vi "gearMiddlePeg.vi"   [LabVIEW 2016]
uses:
  <vilib>/Rock Robotics/WPI/Solenoid/WPI_SolenoidValue.ctl
  <vilib>/Rock Robotics/WPI/Solenoid/WPI_SolenoidSetEnum.vi
types:
  T1 = typedef "WPI_SolenoidValue.ctl" = enum16{"Off", "On", "Forward", "Reverse"}
  T2 = typedef "WPI_MotorControlDeviceRef.ctl" = cluster{"DeviceStatus":errorcluster, "Type":T3, "PWM":cluster{"PWM Channel":T4, "DeadBand":T5}, "CAN":cluster{"Device Number":u8, "SetOutput VI Ref":variant, "GetOutput VI Ref":variant, "Enable VI Ref":variant, "Disable VI Ref":variant, "Data":variant}, "Invert":bool}
  T3 = typedef "WPI_MotorControlType.ctl" = enum16{"PWM", "CAN"}
  T4 = typedef "FPGA_DIOPWMChannel.ctl" = enum8{"PWM 0", "PWM 1", "PWM 2", "PWM 3", "PWM 4", "PWM 5", "PWM 6", "PWM 7", "PWM 8", "PWM 9", "PWM MXP 0", "PWM MXP 1", "PWM MXP 2", "PWM MXP 3", "PWM MXP 4", "PWM MXP 5", "PWM MXP 6", "PWM MXP 7", "PWM MXP 8", "PWM MXP 9", "Invalid"}
  T5 = typedef "WPI_PWMDeadband.ctl" = cluster{"Name":string, "maxPositivePwm":i32, "minPositivePwm":i32, "centerPwm":i32, "maxNegativePwm":i32, "minNegativePwm":i32, "angularRange":u16}
  T6 = typedef "WPI_SolenoidDevRef.ctl" = cluster{"DevStatus":errorcluster, "Pneumatics Control Module":u8, "Forward Solenoid Channel":T7, "Reverse Solenoid Channel":T7}
  T7 = typedef "WPI_SolenoidChannel.ctl" = enum8{"Solenoid 0", "Solenoid 1", "Solenoid 2", "Solenoid 3", "Solenoid 4", "Solenoid 5", "Solenoid 6", "Solenoid 7", "Invalid"}
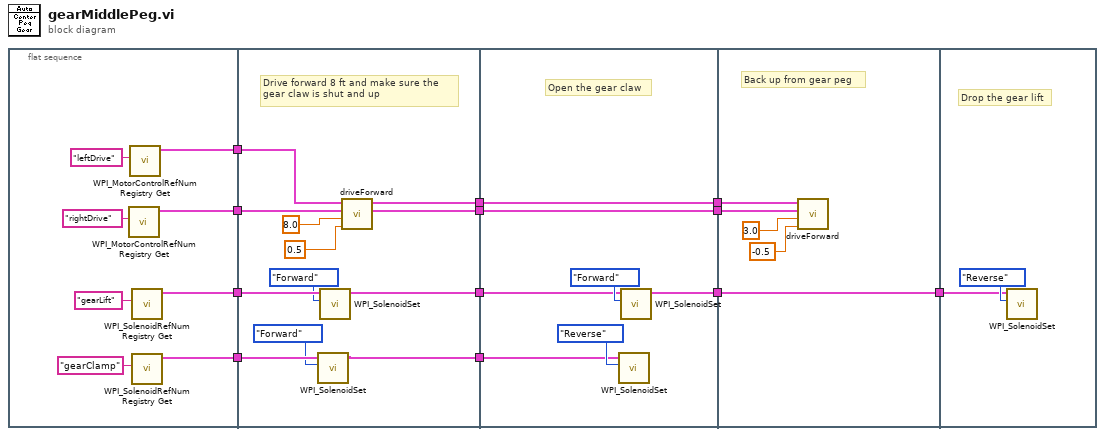
[diagram p0: block diagram]
diagram:
  n1 = flat-sequence {
    tunnel: [w16] -> w12
    tunnel: [w15] -> w11
    tunnel: [w14] -> w10
    tunnel: [w13] -> w9
    tunnel: w12 -> [w32]
    tunnel: w11 -> [w31]
    tunnel: w10 -> [w28]
    tunnel: w9 -> [w27]
    tunnel: [w24] -> w8
    tunnel: [w23] -> w7
    tunnel: [w22] -> w5
    tunnel: [w21] -> w4
    tunnel: w8 -> [w37]
    tunnel: w7 -> [w36]
    tunnel: [w35] -> w6
    tunnel: w5 -> [w35]
    tunnel: w4 -> [w34]
    tunnel: [w34] -> w3
    tunnel: [w33] -> w1
    tunnel: w6 -> [w44]
    tunnel: w3 -> [w43]
    tunnel: [w40] -> w2
    tunnel: w1 -> [w40]
    tunnel: w2 -> [w45]
    frame #0 {
      n2 = call <vilib>:"WPI_MotorControlRefNum Registry Get.vi"("refnum name"="rightDrive") -> ("MotorControlDevRef"=w15:T2)  [unwired: 9 in, 1 out]
      n3 = call <vilib>:"WPI_MotorControlRefNum Registry Get.vi"("refnum name"="leftDrive") -> ("MotorControlDevRef"=w16:T2)  [unwired: 9 in, 1 out]
      n4 = call <vilib>:"WPI_SolenoidRefNum Registry Get.vi"("refnum name"="gearLift") -> ("SolenoidDevRef"=w14:T6)  [unwired: 9 in, 1 out]
      n5 = call <vilib>:"WPI_SolenoidRefNum Registry Get.vi"("refnum name"="gearClamp") -> ("SolenoidDevRef"=w13:T6)  [unwired: 9 in, 1 out]
    }
    frame #1 {
      # "Drive forward 8 ft and make sure the \ngear claw is shut and up"
      n6 = call-poly <vilib>:"WPI_SolenoidSet.vi"("Value"=WPI_SolenoidValue."Forward", "SolenoidDevRef"=w27) -> ("SolenoidDevRef"=w23:T6)  [unwired: 8 in, 1 out]
      n7 = call-poly <vilib>:"WPI_SolenoidSet.vi"("Value"=WPI_SolenoidValue."Forward", "SolenoidDevRef"=w28) -> ("SolenoidDevRef"=w24:T6)  [unwired: 8 in, 1 out]
      n8 = call "driveForward.vi"("speed (%)"=0.5 ("distance (ft)"), "distance (ft)"=8.0, "rightMotor"=w31, "leftMotor"=w32) -> ("rightMotor"=w21:T2, "leftMotor"=w22:T2)  [unwired: 6 in]
    }
    frame #2 {
      # "Open the gear claw"
      n9 = call-poly <vilib>:"WPI_SolenoidSet.vi"("Value"=WPI_SolenoidValue."Reverse", "SolenoidDevRef"=w36) -> ()  [unwired: 8 in, 2 out]
      n10 = call-poly <vilib>:"WPI_SolenoidSet.vi"("Value"=WPI_SolenoidValue."Forward", "SolenoidDevRef"=w37) -> ("SolenoidDevRef"=w33:T6)  [unwired: 8 in, 1 out]
    }
    frame #3 {
      # "Back up from gear peg"
      n11 = call "driveForward.vi"("speed (%)"=-0.5, "distance (ft)"=3.0, "rightMotor"=w43, "leftMotor"=w44) -> ()  [unwired: 6 in, 2 out]
    }
    frame #4 {
      # "Drop the gear lift"
      n12 = call-poly <vilib>:"WPI_SolenoidSet.vi"("Value"=WPI_SolenoidValue."Reverse", "SolenoidDevRef"=w45) -> ()  [unwired: 8 in, 2 out]
    }
  }
